vi "SELECT LIMITES FROM OP100Limites.vi"(8 "errin":errorcluster, 10 "30%                                  70% 2":bool, 11 "type":string) -> (0 "error out":errorcluster, 2 "données":string[](array[string]), 3 "data":T1)   [LabVIEW 2020]
doc: "Récupère les limites de test"
uses:
  subVI/Ctrl/L2T.ctl
  subVI/VarGLO/Global var.vi
  <vilib>/addons/database/Connection.llb/DB Tools Open Connec (String).vi
  <vilib>/addons/database/Connection.llb/Conn Execute.vi
  <vilib>/addons/database/Recordset.llb/Rec Fetch Recordset Data (R).vi
  subVI/VarGLO/Global Limite de test.vi
  <vilib>/addons/database/Recordset.llb/Rec Destroy - Connection.vi
  <vilib>/addons/database/NI_Database_API.lvlib
panel:
  out "recordset data":variant[][](array[variant])
  # "Pre DCIR_____________________________________"
  # "intra DCIR_____________________________________"
  # "Post DCIR_____________________________________"
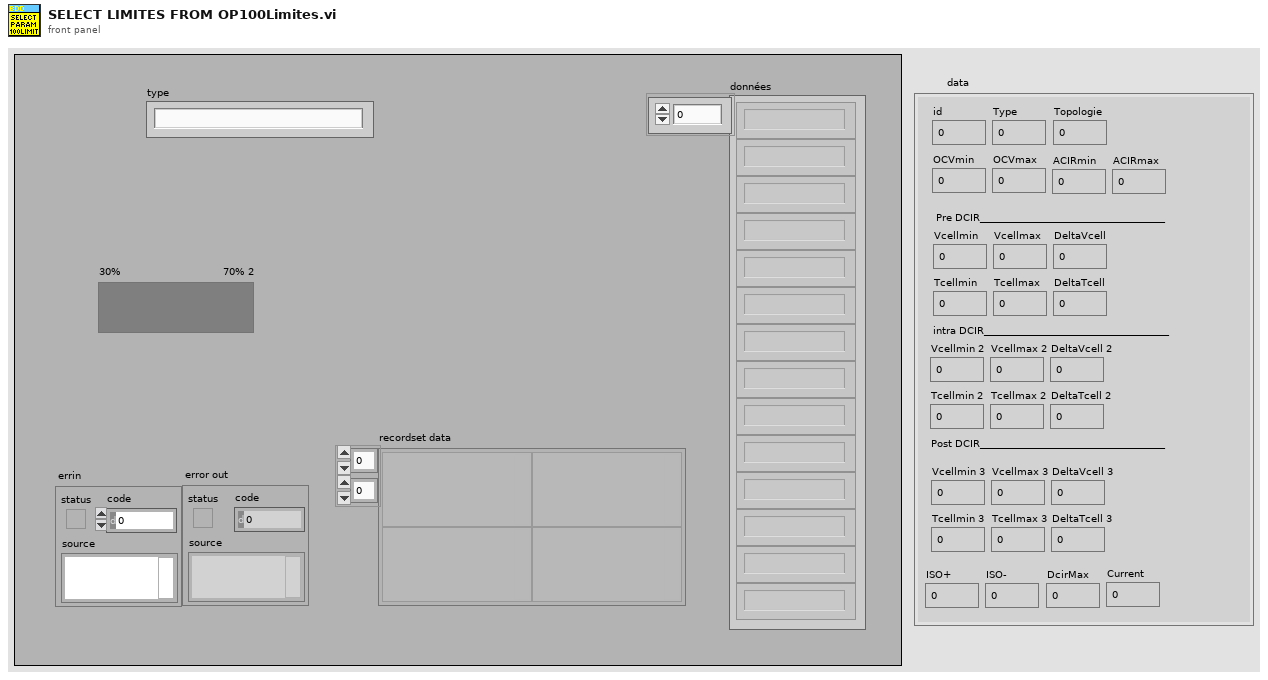
[diagram p1: front panel]
types:
  T1 = typedef "L2T.ctl" = cluster{"id":dbl, "Type":dbl, "OCVmin":dbl, "OCVmax":dbl, "ACIRmin":dbl, "ACIRmax":dbl, "Vcellmin":dbl, "Vcellmax":dbl, "DeltaVcell":dbl, "Tcellmin":dbl, "Tcellmax":dbl, "DeltaTcell":dbl, "ISO+":dbl, "ISO-":dbl, "DcirMax":dbl, "Current":dbl, "Topologie":dbl, "Vcellmin 2":dbl, "Vcellmax 2":dbl, "DeltaVcell 2":dbl, "Tcellmin 2":dbl, "Tcellmax 2":dbl, "DeltaTcell 2":dbl, "Vcellmin 3":dbl, "Vcellmax 3":dbl, "DeltaVcell 3":dbl, "Tcellmin 3":dbl, "Tcellmax 3":dbl, "DeltaTcell 3":dbl}
  T2 = typedef "NI_Database_API.lvlib/Conn ObjectReference.ctl" = refnum<k1>
  T3 = typedef "NI_Database_API.lvlib/Rec ObjectReference.ctl" = refnum<k1>
  T4 = cluster{"[0]":dbl, "[1]":dbl, "[2]":dbl, "[3]":dbl, "[4]":dbl, "[5]":dbl, "[6]":dbl, "[7]":dbl, "[8]":dbl, "[9]":dbl, "[10]":dbl, "[11]":dbl, "[12]":dbl, "[13]":dbl, "[14]":dbl, "[15]":dbl, "[16]":dbl, "[17]":dbl, "[18]":dbl, "[19]":dbl, "[20]":dbl, "[21]":dbl, "[22]":dbl, "[23]":dbl, "[24]":dbl, "[25]":dbl, "[26]":dbl, "[27]":dbl, "[28]":dbl}
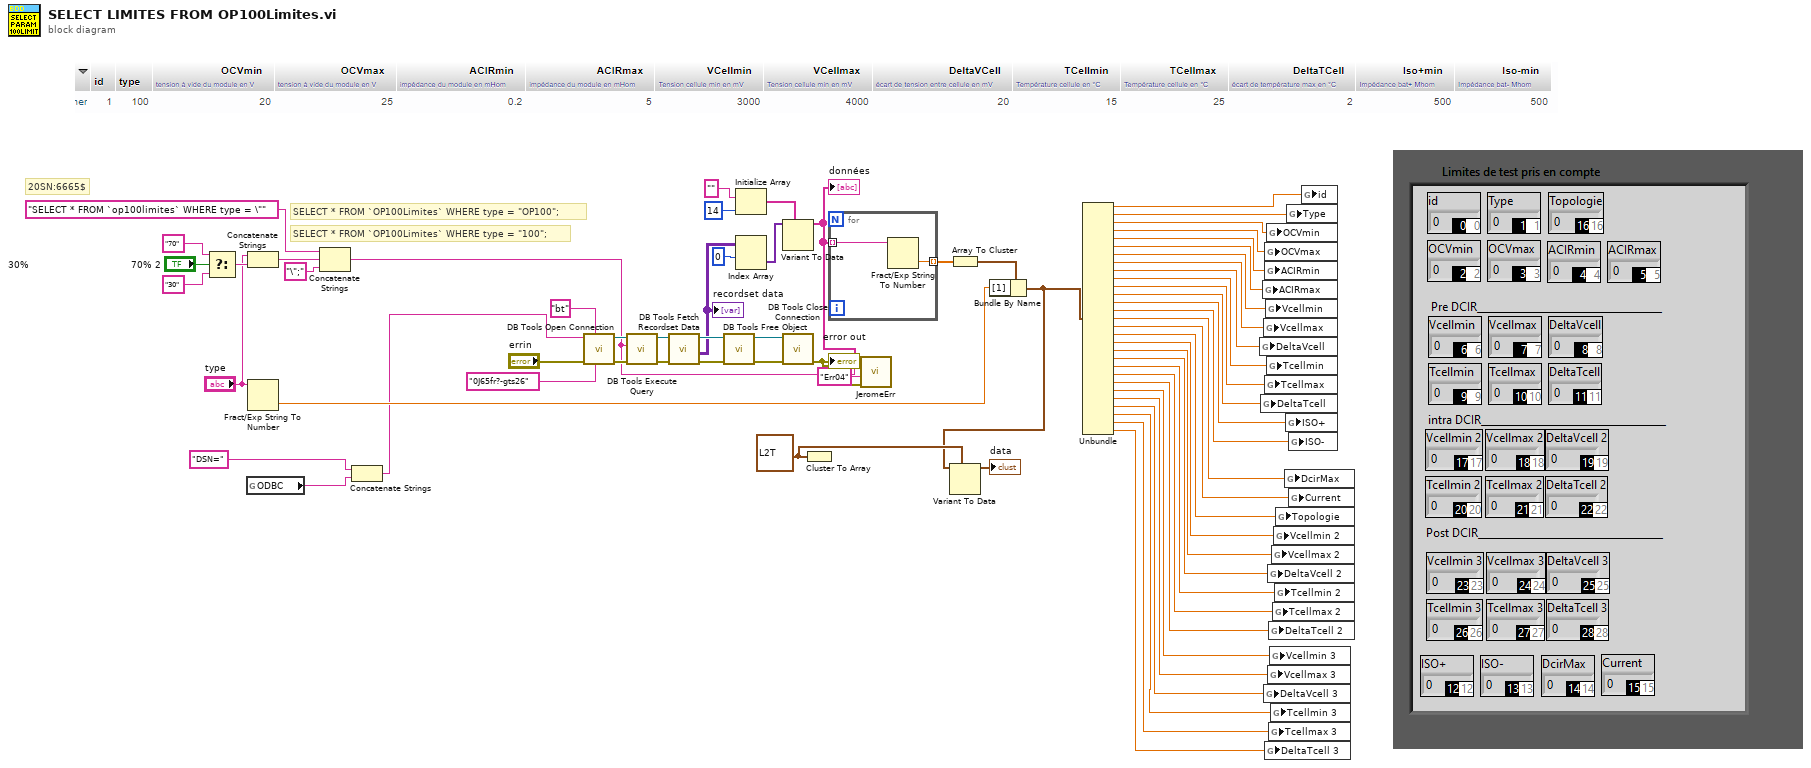
[diagram p0: block diagram]
diagram:
  w7 = T1 {"id"=0.0, "Type"=0.0, "OCVmin"=0.0, "OCVmax"=0.0, "ACIRmin"=0.0, "ACIRmax"=0.0, "Vcellmin"=0.0, "Vcellmax"=0.0, "DeltaVcell"=0.0, "Tcellmin"=0.0, "Tcellmax"=0.0, "DeltaTcell"=0.0, "ISO+"=0.0, "ISO-"=0.0, "DcirMax"=0.0, "Current"=0.0, "Topologie"=0.0, "Vcellmin 2"=0.0, "Vcellmax 2"=0.0, "DeltaVcell 2"=0.0, "Tcellmin 2"=0.0, "Tcellmax 2"=0.0, "DeltaTcell 2"=0.0, "Vcellmin 3"=0.0, "Vcellmax 3"=0.0, "DeltaVcell 3"=0.0, "Tcellmin 3"=0.0, "Tcellmax 3"=0.0, "DeltaTcell 3"=0.0} ("L2T")
  # "SELECT * FROM `OP100Limites` WHERE type = \"OP100\";"
  # "SELECT * FROM `OP100Limites` WHERE type = \"100\";"
  # "20SN:6665$"
  n1 = Select ("Sélectionner")(t="70", s="30%                                  70% 2", f="30" ("cas faux")) -> (s? t:f=w43:string)
  n2 = global read "Global var.vi" "ODBC"() -> (w2:string)
  n3 = Concatenate Strings("type", w43) -> (w42:string)
  n4 = Fract/Exp String To Number(string="type") -> (number=w47:dbl)  [unwired: 3 in, 1 out]
  n5 = Concatenate Strings("SELECT * FROM `op100limites` WHERE type = \"" ("SQL query"), w42, "\";" ("chaîne")) -> (w38:string)
  n6 = Concatenate Strings("DSN=", w2) -> (w1:string)
  n7 = call-poly <vilib>:"DB Tools Open Connection.vi"("password"="0J65fr?-gts26", "userID"="bt", "error in (no error)"="errin", "connection information"=w1) -> ("error out"=w67:errorcluster, "connection reference"=w65:T2)  [unwired: 4 in]
  n8 = call-poly <vilib>:"DB Tools Execute Query.vi"("error in (no error)"=w67, "SQL query"=w38, "connection reference"=w65) -> ("error out"=w61:errorcluster, "recordset reference"=w60:T3)  [unwired: 5 in]
  n9 = call-poly <vilib>:"DB Tools Fetch Recordset Data.vi"("error in (no error)"=w61, "recordset reference"=w60) -> ("error out"=w62:errorcluster, "recordset data"=w55:variant[][], "recordset reference out"=w59:T3)  [unwired: 3 in]
  "recordset data" <- w55
  n10 = call-poly <vilib>:"DB Tools Free Object.vi"("error in (no error)"=w62, "recordset reference"=w59) -> ("error out"=w66:errorcluster, "connection reference"=w64:T2)  [unwired: 8 in]
  n11 = Initialize Array("", 14 ("taille de la dimension")) -> (w51:string[])
  n12 = Index Array(array=w55, index (row)=0 ("indice (ligne)")) -> (element=w53:variant[])  [unwired: 1 in]
  n13 = Variant To Data ("Variant en donnée")(type=w51, Variant=w53) -> (data=w39:string[])  [unwired: 1 in, 1 out]
  "données" <- w39
  n14 = call <vilib>:"DB Tools Close Connection.vi"("error in (no error)"=w66, "connection reference"=w64) -> ("error out"=w40:errorcluster)  [unwired: 5 in]
  "error out" <- w40
  n15 = Cluster To Array(cluster=w7) -> ()  [unwired: 1 out]
  n16 = for {
    tunnel: w39 -> [w69] mode=indexing
    tunnel: [w68] -> w50 mode=indexing
    n17 = Fract/Exp String To Number(string=w69) -> (number=w68:dbl)  [unwired: 3 in, 1 out]
  }
  n18 = call "JeromeErr.vi"("Errin"=w40, "CodeERR"="Err04", "RequetteSQL"=w38, "RetourSQL"=w39) -> ()  [unwired: 8 in]
  n19 = Array To Cluster ("Tableau en cluster")(array=w50) -> (cluster=w6:T4)
  n20 = Bundle By Name(cluster=w6, "[1]"=w47) -> (w4:T4)
  n21 = Variant To Data(type=w7, Variant=w4) -> (data=→"data":T1)  [unwired: 1 in, 1 out]
  n22 = Unbundle(w4) -> ("[0]"=w36:dbl, "[1]"=w35:dbl, "[2]"=w34:dbl, "[3]"=w33:dbl, "[4]"=w32:dbl, "[5]"=w31:dbl, "[6]"=w30:dbl, "[7]"=w29:dbl, "[8]"=w28:dbl, "[9]"=w27:dbl, "[10]"=w26:dbl, "[11]"=w25:dbl, "[12]"=w24:dbl, "[13]"=w23:dbl, "[14]"=w22:dbl, "[15]"=w21:dbl, "[16]"=w20:dbl, "[17]"=w19:dbl, "[18]"=w18:dbl, "[19]"=w17:dbl, "[20]"=w16:dbl, "[21]"=w15:dbl, "[22]"=w14:dbl, "[23]"=w13:dbl, "[24]"=w12:dbl, "[25]"=w11:dbl, "[26]"=w10:dbl, "[27]"=w9:dbl, "[28]"=w8:dbl)
  n23 = global write "Global Limite de test.vi" "DeltaVcell"(w28) -> ()
  n24 = global write "Global Limite de test.vi" "DeltaTcell"(w25) -> ()
  n25 = global write "Global Limite de test.vi" "ACIRmax"(w31) -> ()
  n26 = global write "Global Limite de test.vi" "Vcellmax"(w29) -> ()
  n27 = global write "Global Limite de test.vi" "DeltaVcell 3"(w11) -> ()
  n28 = global write "Global Limite de test.vi" "OCVmax"(w33) -> ()
  n29 = global write "Global Limite de test.vi" "ACIRmin"(w32) -> ()
  n30 = global write "Global Limite de test.vi" "Tcellmax"(w26) -> ()
  n31 = global write "Global Limite de test.vi" "DeltaTcell 3"(w8) -> ()
  n32 = global write "Global Limite de test.vi" "Vcellmin"(w30) -> ()
  n33 = global write "Global Limite de test.vi" "OCVmin"(w34) -> ()
  n34 = global write "Global Limite de test.vi" "Tcellmin"(w27) -> ()
  n35 = global write "Global Limite de test.vi" "DeltaVcell 2"(w17) -> ()
  n36 = global write "Global Limite de test.vi" "Vcellmax 3"(w12) -> ()
  n37 = global write "Global Limite de test.vi" "DeltaTcell 2"(w14) -> ()
  n38 = global write "Global Limite de test.vi" "Tcellmax 3"(w9) -> ()
  n39 = global write "Global Limite de test.vi" "Vcellmin 3"(w13) -> ()
  n40 = global write "Global Limite de test.vi" "Tcellmin 3"(w10) -> ()
  n41 = global write "Global Limite de test.vi" "Vcellmax 2"(w18) -> ()
  n42 = global write "Global Limite de test.vi" "Tcellmax 2"(w15) -> ()
  n43 = global write "Global Limite de test.vi" "Vcellmin 2"(w19) -> ()
  n44 = global write "Global Limite de test.vi" "Tcellmin 2"(w16) -> ()
  n45 = global write "Global Limite de test.vi" "Topologie"(w20) -> ()
  n46 = global write "Global Limite de test.vi" "DcirMax"(w22) -> ()
  n47 = global write "Global Limite de test.vi" "ISO+"(w24) -> ()
  n48 = global write "Global Limite de test.vi" "Type"(w35) -> ()
  n49 = global write "Global Limite de test.vi" "ISO-"(w23) -> ()
  n50 = global write "Global Limite de test.vi" "Current"(w21) -> ()
  n51 = global write "Global Limite de test.vi" "id"(w36) -> ()
